vi "Get Bus Controller and Remote Terminals Handles from BTI Channel.vi"(8 "error in":errorcluster, 10 "terminal addresses":T1[](array[typedef]), 11 "channel handle in":u64) -> (0 "error out":errorcluster, 1 "remote terminal handles out":u64[](array[numeric]), 2 "bus controller handle out":u64, 3 "channel handle out":u64)   [LabVIEW 2020, in "AIM MIL-STD-1553 Engine.lvlib" / "Custom Device.lvlib"]
uses:
  Custom Device.lvlib
  Shared/Address.ctl
  <instrlib>/BTI1553Lib/BTI1553LV.lvlib
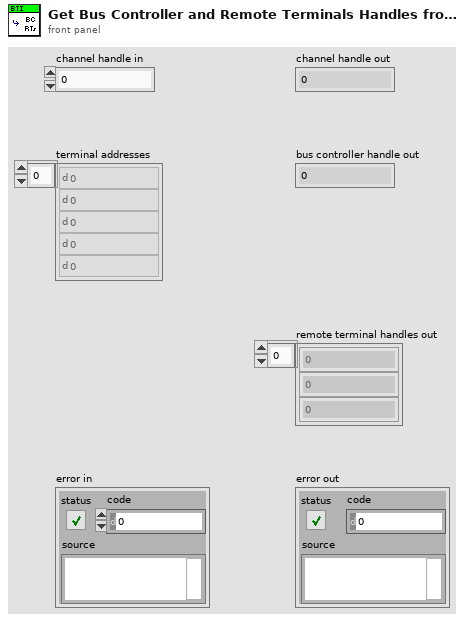
[diagram p1: front panel]
types:
  T1 = typedef "Address.ctl" = u16
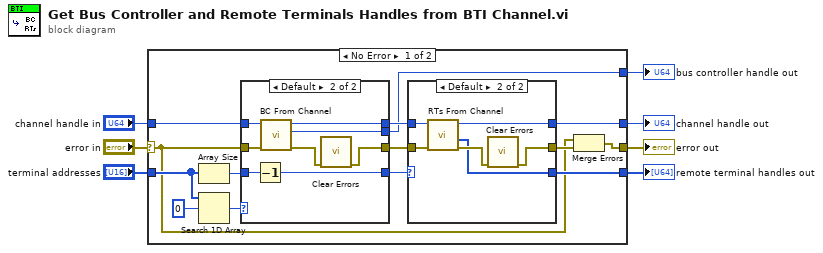
[diagram p0: block diagram]
diagram:
  n1 = case shown="No Error" "error in" {
    selector: "error in" -> [w8 w41]
    tunnel: "channel handle in" -> [w20 w42]
    tunnel: [w9 w41] -> w5
    tunnel: [w19 w42] -> w4
    tunnel: "terminal addresses" -> [w15 _]
    tunnel: [w16 _] -> w2
    tunnel: [w10 _] -> w1
    frame No Error {
      n2 = Array Size(array=w15) -> (size(s)=w14:i32)
      n3 = Search 1D Array(1D array=w15, element=T1 0) -> (index of element=w17:i32)  [unwired: 1 in]
      n4 = case shown="Default" w17 {
        tunnel: [w32 w40] -> w21
        tunnel: w20 -> [w32 w39]
        tunnel: w8 -> [w31 w38]
        tunnel: [w31 w33] -> w11
        tunnel: [_ w36] -> w16
        tunnel: w14 -> [w30 w35]
        tunnel: [w30 w34] -> w13
        frame -1 {
        }
        frame Default {
          n5 = Decrement(x=w35) -> (x-1=w34:i32)
          n6 = call <instrlib>:"BC From Channel.vi"("error in (no error)"=w38, "channel handle in"=w39) -> ("error out"=w37:errorcluster, "bus controller handle out"=w36:u64, "channel handle out"=w40:u64)  [unwired: 7 in]
          n7 = call <vilib>:"Clear Errors.vi"("error in (no error)"=w37) -> ("error out"=w33:errorcluster)  [unwired: 5 in, 1 out]
        }
      }
      n8 = case shown="Default" w13 {
        tunnel: w21 -> [w23 w29]
        tunnel: [w23 w28] -> w19
        tunnel: [w22 w24] -> w12
        tunnel: w11 -> [w22 w27]
        tunnel: [_ w25] -> w10
        frame ..0 {
        }
        frame Default {
          n9 = call <instrlib>:"RTs From Channel.vi"("error in (no error)"=w27, "channel handle in"=w29) -> ("error out"=w26:errorcluster, "remote terminal handles out"=w25:u64[], "channel handle out"=w28:u64)  [unwired: 6 in, 1 out]
          n10 = call <vilib>:"Clear Errors.vi"("error in (no error)"=w26) -> ("error out"=w24:errorcluster)  [unwired: 5 in, 1 out]
        }
      }
      n11 = Merge Errors(w8, w12) -> (w9:errorcluster)
    }
    frame Error {
    }
  }
  "bus controller handle out" <- w2
  "remote terminal handles out" <- w1
  "error out" <- w5
  "channel handle out" <- w4
